vi "FGV_UIchange.vi"(7 "Enum":T1, 8 "error in (no error)":errorcluster, 9 "Modules":string[](array[string])=["PXI6251_ai.vi"], 10 "UIname":string="PXI8431_7_com_slot7.vi", 11 "ModulesPath":path) -> (0 "error out":errorcluster, 2 "UI?":bool, 3 "InsertVI":refnum<vi>)   [LabVIEW 2017]
uses:
  Func_UIchange.ctl
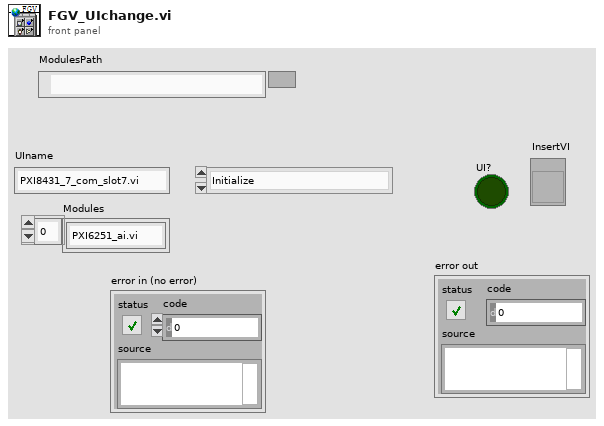
[diagram p1: front panel]
types:
  T1 = typedef "Func_UIchange.ctl" = enum16{"Initialize", "Load Modules", "get UI"}
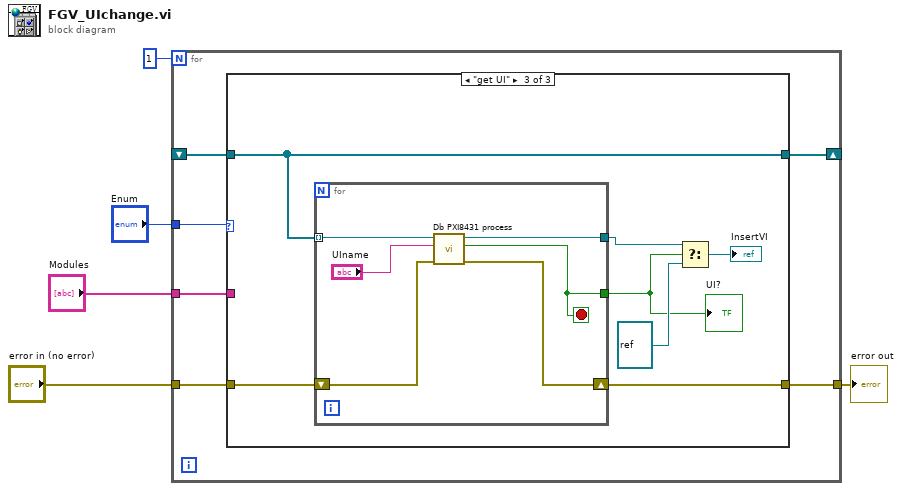
[diagram p0: block diagram]
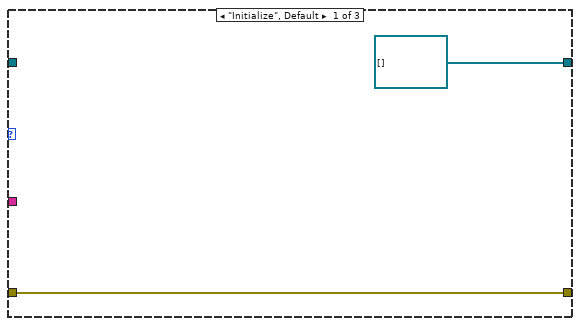
[diagram p2: hidden frame]
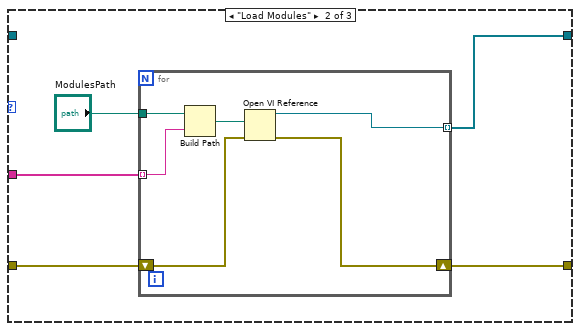
[diagram p3: hidden frame]
diagram:
  n1 = for {
    N: 1 -> [_]
    shift-right: [w8] -> _
    shift-left: _ -> [w6]
    tunnel: "Enum" -> [w11]
    tunnel: "Modules" -> [w10]
    tunnel: "error in (no error)" -> [w9]
    tunnel: [w7] -> w1
    n2 = case shown="\"get UI\"" w11 {
      tunnel: w10 -> [_ w17 _]
      tunnel: w9 -> [w13 w16 w30]
      tunnel: [refnum<vi>[] [] w15 w31] -> w8
      tunnel: [w13 w14 w29] -> w7
      tunnel: w6 -> [_ _ w31]
      frame "Initialize", Default {
      }
      frame "Load Modules" {
        n3 = for {
          tunnel: "ModulesPath" -> [w24]
          tunnel: w17 -> [w23] mode=indexing
          shift-right: [w20] -> w14
          shift-left: w16 -> [w21]
          tunnel: [w19] -> w15 mode=indexing
          n4 = Build Path(base path=w24, name or relative path=w23) -> (appended path=w22:path)
          n5 = Open VI Reference(vi path=w22, error in (no error)=w21) -> (vi reference=w19:refnum<vi>, error out=w20:errorcluster)  [unwired: 4 in]
        }
      }
      frame "get UI" {
        n6 = for {
          tunnel: w31 -> [w37] mode=indexing
          shift-right: [w32] -> w29
          shift-left: w30 -> [w36]
          tunnel: [w35] -> w26
          tunnel: [w34] -> w25
          stop <- w34 stop-if-true
          n7 = call "Db PXI8431 process.vi"("error in (no error)"=w36, "UIname"="UIname", "VI in"=w37) -> ("error out"=w32:errorcluster, "Boolean"=w34:bool, "VI out"=w35:refnum<vi>)  [unwired: 6 in]
        }
        "UI?" <- w25
        n8 = Select(t=w26, s=w25, f=refnum<vi> refnum) -> (s? t:f=→"InsertVI":refnum<vi>)
      }
    }
  }
  "error out" <- w1
